vi "HWE Url--constant.vi"() -> (3 "url":string)   [LabVIEW 2025]
doc: "URL of hasbun-wood-engineering (used to create a hyperlink)."
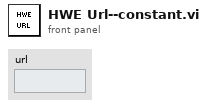
[diagram p1: front panel]
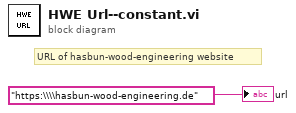
[diagram p0: block diagram]
diagram:
  # "URL of hasbun-wood-engineering website"
  "url" <- "https:\\\\hasbun-wood-engineering.de"
